vi "Update(Camera)_v2.vi"(8 "error in (no error)":errorcluster, 10 "Camera_Settings":T2 {"WhiteB." min=2000 max=7500 step=1; "Gain" max=255 step=5; "Exposure" min=0 max=9 step=5; "Focus" step=5}, 11 "Session in":T1) -> (0 "error out":errorcluster, 3 "Session out":T1)   [LabVIEW 2020]
uses:
  Controls/Camera_Settings.ctl
  <vilib>/userDefined/High Color/IMAQdx.ctl
  1c965d0a-2fbf-4a15-954e-c94853878a6e.vi
  5c231780-0e81-4dfd-8826-f815c49f2449.vi
  <resource>/objmgr/imaqdx.rc
  <vilib>/vision/driver/NI_Vision_Acquisition_Software.lvlib
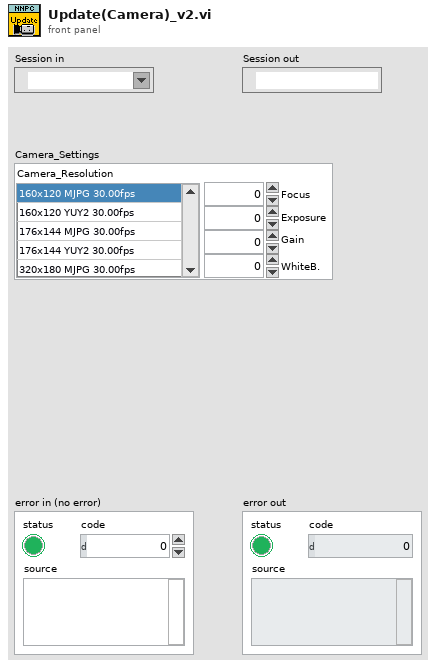
[diagram p1: front panel]
types:
  T1 = typedef "IMAQdx.ctl" = refnum<k21>
  T2 = typedef "Camera_Settings.ctl" = cluster{"Camera_Resolution":i32, "Focus":u8, "Exposure":i32, "Gain":u32, "WhiteB.":i32}
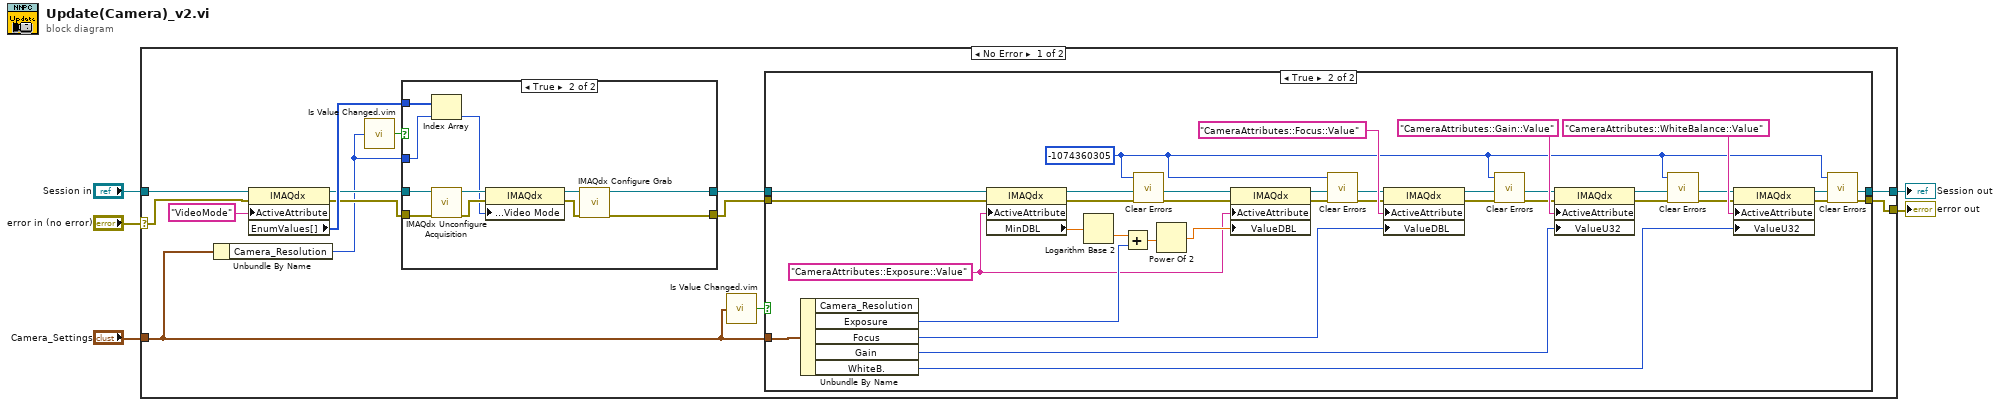
[diagram p0: block diagram]
diagram:
  n1 = case shown="No Error" "error in (no error)" {
    selector: "error in (no error)" -> [w17 w67]
    tunnel: "Session in" -> [w18 w66]
    tunnel: "Camera_Settings" -> [w7 _]
    tunnel: [w10 w66] -> w2
    tunnel: [w9 w67] -> w1
    frame No Error {
      n2 = Unbundle By Name(w7) -> ("Camera_Resolution"=w8:i32)
      n3 = property class="IMAQdx"(reference=w18, error in=w17, "ActiveAttribute"="VideoMode") -> (reference out=w15:T1, error out=w14:errorcluster, "EnumValues[]"=w16:u32[])
      n4 = call "Is Value Changed.vim"("value"=w8) -> ("changed or first call?"=w19:bool)
      n5 = case shown="True" w19 {
        tunnel: [w21 w23] -> w12
        tunnel: [w20 w22] -> w11
        tunnel: w16 -> [_ w32]
        tunnel: w8 -> [_ w31]
        tunnel: w14 -> [w20 w25]
        tunnel: w15 -> [w21 w24]
        frame False {
        }
        frame True {
          n6 = Index Array(array=w32, index=w31) -> (element=w26:u32)
          n7 = call <vilib>:"IMAQdx Unconfigure Acquisition.vi"("error in"=w25, "Session In"=w24) -> ("error out"=w27:errorcluster, "Session Out"=w30:T1)  [unwired: 8 out]
          n8 = property class="IMAQdx"(reference=w30, error in=w27, "Acquisition Attributes:Video Mode"=w26) -> (reference out=w29:T1, error out=w28:errorcluster)
          n9 = call <vilib>:"IMAQdx Configure Grab.vi"("error in"=w28, "Session In"=w29) -> ("error out"=w22:errorcluster, "Session Out"=w23:T1)  [unwired: 2 in, 6 out]
        }
      }
      n10 = call "Is Value Changed.vim"("value"=w7) -> ("changed or first call?"=w6:bool)
      n11 = case shown="True" w6 {
        tunnel: w12 -> [w34 w62]
        tunnel: w11 -> [w33 w61]
        tunnel: [w34 w44] -> w10
        tunnel: [w33 w42] -> w9
        tunnel: w7 -> [_ w36]
        frame False {
        }
        frame True {
          w35 = "CameraAttributes::Exposure::Value" ("ActiveAttribute")
          w37 = -1074360305 ("specific error code to clear (0: all)")
          n12 = Unbundle By Name(w36) -> ("Exposure"=w65:i32, "Focus"=w55:u8, "Gain"=w52:u32, "WhiteB."=w49:i32)  [unwired: 1 out]
          n13 = property class="IMAQdx"(reference=w62, error in=w61, "ActiveAttribute"=w35) -> (reference out=w48:T1, error out=w59:errorcluster, "MinDBL"=w60:dbl)
          n14 = Logarithm Base 2(1:w60) -> (0:w63:dbl)
          n15 = Add(x=w63, y=w65) -> (x+y=w64:dbl)
          n16 = call <vilib>:"Clear Errors.vi"("error in (no error)"=w59, "specific error code to clear (0: all)"=w37) -> ("error out"=w38:errorcluster)  [unwired: 4 in, 1 out]
          n17 = Power Of 2(x=w64) -> (2^x=w58:dbl)
          n18 = property class="IMAQdx"(reference=w48, error in=w38, "ActiveAttribute"=w35, "ValueDBL"=w58) -> (reference out=w47:T1, error out=w56:errorcluster)
          n19 = call <vilib>:"Clear Errors.vi"("error in (no error)"=w56, "specific error code to clear (0: all)"=w37) -> ("error out"=w39:errorcluster)  [unwired: 4 in, 1 out]
          n20 = property class="IMAQdx"(reference=w47, error in=w39, "ActiveAttribute"="CameraAttributes::Focus::Value", "ValueDBL"=w55) -> (reference out=w46:T1, error out=w53:errorcluster)
          n21 = call <vilib>:"Clear Errors.vi"("error in (no error)"=w53, "specific error code to clear (0: all)"=w37) -> ("error out"=w40:errorcluster)  [unwired: 4 in, 1 out]
          n22 = property class="IMAQdx"(reference=w46, error in=w40, "ActiveAttribute"="CameraAttributes::Gain::Value", "ValueU32"=w52) -> (reference out=w45:T1, error out=w50:errorcluster)
          n23 = call <vilib>:"Clear Errors.vi"("error in (no error)"=w50, "specific error code to clear (0: all)"=w37) -> ("error out"=w41:errorcluster)  [unwired: 4 in, 1 out]
          n24 = property class="IMAQdx"(reference=w45, error in=w41, "ActiveAttribute"="CameraAttributes::WhiteBalance::Value", "ValueU32"=w49) -> (reference out=w44:T1, error out=w43:errorcluster)
          n25 = call <vilib>:"Clear Errors.vi"("error in (no error)"=w43, "specific error code to clear (0: all)"=w37) -> ("error out"=w42:errorcluster)  [unwired: 4 in, 1 out]
        }
      }
    }
    frame Error {
    }
  }
  "Session out" <- w2
  "error out" <- w1
